vi "GetFileInfoReference.vi"(8 "error in (no error)":errorcluster, 11 "VI in":refnum<vi>) -> (0 "error out":errorcluster, 1 "File Close Action Refnum":refnum<vi>, 2 "File info Refnum":refnum<vi>, 3 "VI out":refnum<vi>, 4 "Master Slave Control":refnum<vi>)   [LabVIEW 2018]
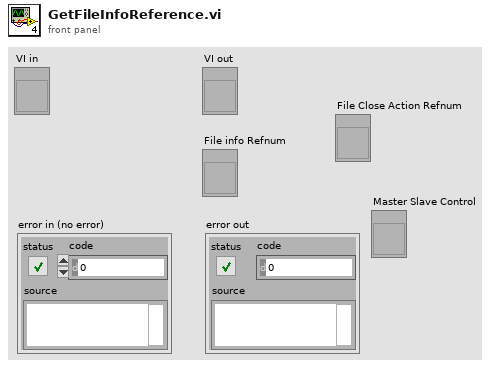
[diagram p1: front panel]
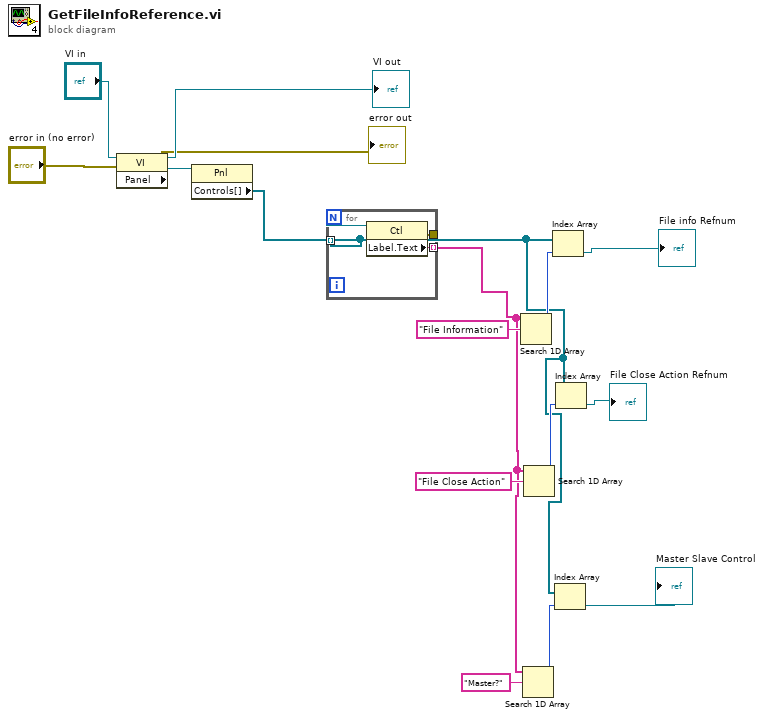
[diagram p0: block diagram]
diagram:
  n1 = property class="VI"(reference="VI in", error in="error in (no error)") -> (reference out=→"VI out":refnum<vi>, error out=→"error out":errorcluster, "Panel"=w11:refnum<vi>)
  n2 = property class="Pnl"(reference=w11) -> ("Controls[]"=w1:refnum<vi>[])  [unwired: 1 in, 2 out]
  n3 = for {
    tunnel: w1 -> [w19] mode=indexing
    tunnel: [w18] -> w3 mode=indexing
    tunnel: [w17] -> _
    n4 = property class="Ctl"(reference=w19) -> (error out=w17:errorcluster, "Label.Text"=w18:string)  [unwired: 1 in, 1 out]
  }
  n5 = Search 1D Array(1D array=w3, element="File Information") -> (index of element=w12:i32)  [unwired: 1 in]
  n6 = Search 1D Array(1D array=w3, element="Master?") -> (index of element=w5:i32)  [unwired: 1 in]
  n7 = Search 1D Array(1D array=w3, element="File Close Action") -> (index of element=w7:i32)  [unwired: 1 in]
  n8 = Index Array(array=w1, index=w12) -> (element=→"File info Refnum":refnum<vi>)
  n9 = Index Array(array=w1, index=w5) -> (element=→"Master Slave Control":refnum<vi>)
  n10 = Index Array(array=w1, index=w7) -> (element=→"File Close Action Refnum":refnum<vi>)
